vi "Write Scale Scale Fit.vi"(6 "Control Ref Queue":T1, 8 "error in (no error)":errorcluster, 9 "Index":i32, 10 "Scale Fit":u8, 11 "2D Plot.lvclass in":refnum<class "2D Plot.lvclass">) -> (0 "error out":errorcluster, 3 "2D Plot.lvclass out":refnum<class "2D Plot.lvclass">)   [LabVIEW 2017, in "2D Plot.lvclass"]
uses:
  <vilib>/Math Plots/2D Math Plots/2D Plot/2D Plot/2D Plot.lvclass
  <vilib>/Math Plots/2D Math Plots/2D Plot/Action String/2DMathPlot Ctrl Act Queue.ctl
  <vilib>/Math Plots/2D Math Plots/2D Plot/Action String/2DMathPlot Ctrl Act Cluster.ctl
  <vilib>/Math Plots/2D Math Plots/2D Plot/Action String/2DMathPlot State Class.ctl
  <vilib>/Math Plots/2D Math Plots/2D Plot/2D Plot/2D Plot.lvclass/2D Plot.ctl
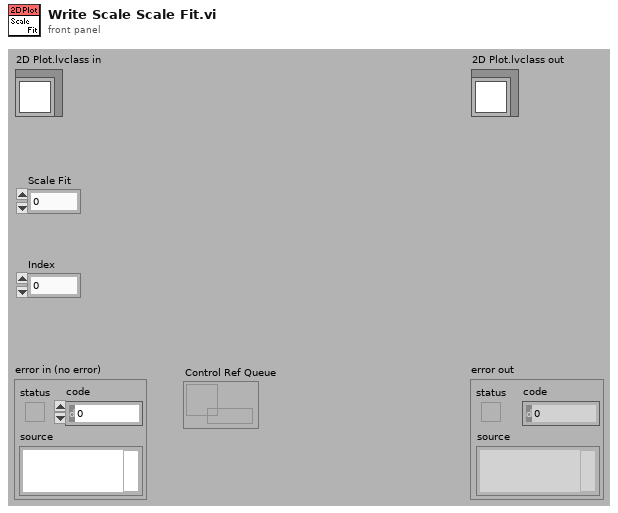
[diagram p1: front panel]
types:
  T1 = typedef "2DMathPlot Ctrl Act Queue.ctl" = refnum<queue>
  T2 = typedef "2D Plot.lvclass/Scale Array.ctl" = T3[]
  T3 = typedef "2D Plot.lvclass/Scale Cluster.ctl" = cluster{"General":cluster{"Editable":bool, "Flipped":bool, "Mapping Mode":u8, "Visible":bool, "Style":u8, "Scale Fit":u8}, "Offset and Multiplier":T4, "Range":cluster{"Minimum":dbl, "Maximum":dbl, "Increment":dbl, "Minor Increment":dbl, "Start":dbl}, "Tick Color":cluster{"Major Color":u32, "Minor Color":u32}, "Gird Color":cluster{"Major Color":u32, "Minor Color":u32}, "Marker":cluster{"Visible":bool, "FG Color":u32, "BG Color":u32, "Font Name":string, "Font Size":u32, "Font Bold":bool, "Font Italic":bool, "Font Strikeout":bool, "Font Underline":bool}, "Name Label":cluster{"Visible":bool, "FG Color":u32, "BG Color":u32, "Font Name":string, "Font Size":u32, "Font Bold":bool, "Font Italic":bool, "Font Strikeout":bool, "Font Underline":bool, "Justification":enum16{"Left", "Center", "Right"}, "Text":string}}
  T4 = typedef "LVOffsetAndMultiplierTypeDef.ctl" = cluster{"Offset":dbl, "Multiplier":dbl}
  T5 = typedef "2DMathPlot Ctrl Act Cluster.ctl" = cluster{"Plot Area Ref":refnum<vi>, "Z Axis Ref":refnum<vi>, "Legend Ref":refnum<vi>, "XControl Ref":refnum<vi>, "Facade Ref":refnum<vi>, "Display State Change Class":T6}
  T6 = typedef "2DMathPlot State Class.ctl" = enum16{"Update All (Undo)", "Update General", "Update Appearance", "Update Format", "Update Scale", "Update Marker", "Update Cursor", "None"}
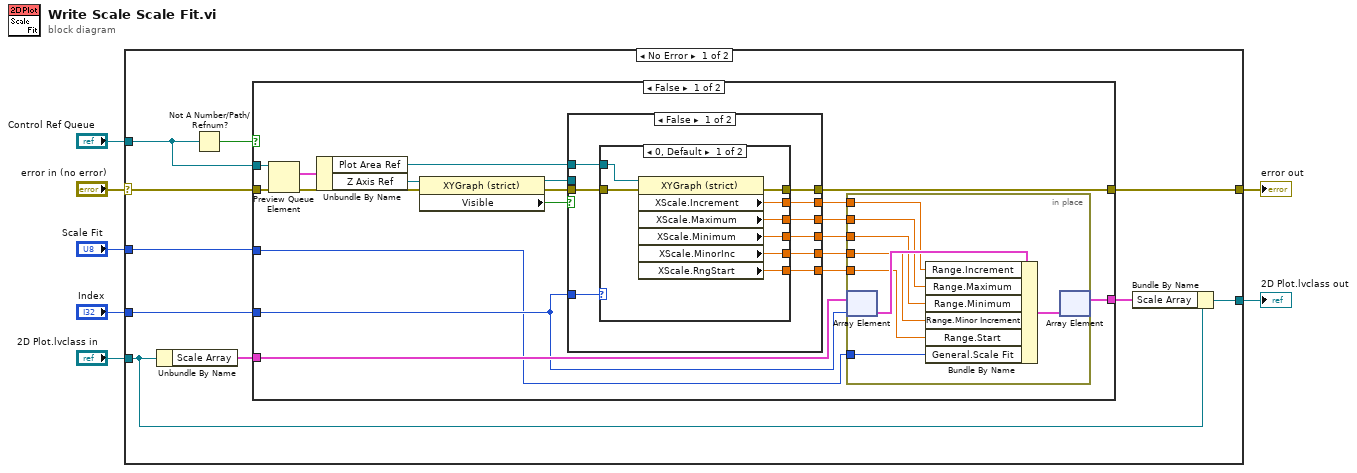
[diagram p0: block diagram]
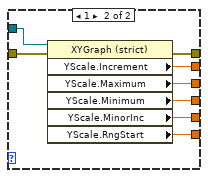
[diagram p2: hidden frame]
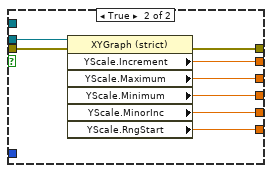
[diagram p3: hidden frame]
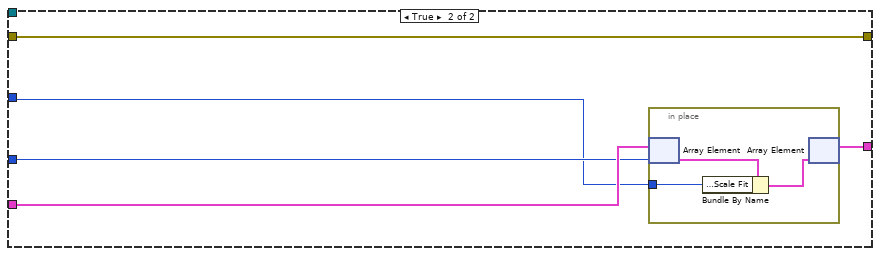
[diagram p4: hidden frame]
diagram:
  n1 = case shown="No Error" "error in (no error)" {
    selector: "error in (no error)" -> [w11 w87]
    tunnel: "2D Plot.lvclass in" -> [w17 w86]
    tunnel: [w16 w86] -> w2
    tunnel: "Control Ref Queue" -> [w9 _]
    tunnel: [w13 w87] -> w1
    tunnel: "Index" -> [w12 _]
    tunnel: "Scale Fit" -> [w10 _]
    frame No Error {
      n2 = Unbundle By Name(w17) -> ("Scale Array"=w15:T2)
      n3 = Not A Number/Path/Refnum?(number/path/refnum=w9) -> (NaN/Path/Refnum?=w8:bool)
      n4 = case shown="False" w8 {
        tunnel: w9 -> [w36 _]
        tunnel: w15 -> [w29 w80]
        tunnel: [w28 w81] -> w14
        tunnel: [w27 w82] -> w13
        tunnel: w12 -> [w21 w79]
        tunnel: w11 -> [w20 w82]
        tunnel: w10 -> [w19 w78]
        frame False {
          n5 = Preview Queue Element(queue=w36, error in (no error)=w20) -> (element=w35:T5, error out=w33:errorcluster)  [unwired: 1 in, 2 out]
          n6 = Unbundle By Name(w35) -> ("Plot Area Ref"=w32:refnum<vi>, "Z Axis Ref"=w18:refnum<vi>)
          n7 = property class="XYGraph (strict)"(reference=w18, error in=w33) -> (reference out=w31:refnum<vi>, error out=w30:errorcluster, "Visible"=w34:bool)
          n8 = case shown="False" w34 {
            tunnel: w30 -> [w53 w76]
            tunnel: [w52 w75] -> w27
            tunnel: w32 -> [w51 _]
            tunnel: w31 -> [_ w77]
            tunnel: [w50 w74] -> w26
            tunnel: [w49 w73] -> w25
            tunnel: [w48 w72] -> w24
            tunnel: [w47 w71] -> w23
            tunnel: [w46 w70] -> w22
            tunnel: w21 -> [w45 _]
            frame False {
              n9 = case shown="0, Default" w45 {
                tunnel: w53 -> [w60 w68]
                tunnel: [w59 w67] -> w52
                tunnel: w51 -> [w61 w69]
                tunnel: [w58 w66] -> w50
                tunnel: [w57 w65] -> w49
                tunnel: [w56 w64] -> w48
                tunnel: [w55 w63] -> w47
                tunnel: [w54 w62] -> w46
                frame 0, Default {
                  n10 = property class="XYGraph (strict)"(reference=w61, error in=w60) -> (error out=w59:errorcluster, "XScale.Increment"=w58:dbl, "XScale.Maximum"=w57:dbl, "XScale.Minimum"=w56:dbl, "XScale.MinorInc"=w55:dbl, "XScale.RngStart"=w54:dbl)  [unwired: 1 out]
                }
                frame 1 {
                  n11 = property class="XYGraph (strict)"(reference=w69, error in=w68) -> (error out=w67:errorcluster, "YScale.Increment"=w66:dbl, "YScale.Maximum"=w65:dbl, "YScale.Minimum"=w64:dbl, "YScale.MinorInc"=w63:dbl, "YScale.RngStart"=w62:dbl)  [unwired: 1 out]
                }
              }
            }
            frame True {
              n12 = property class="XYGraph (strict)"(reference=w77, error in=w76) -> (error out=w75:errorcluster, "YScale.Increment"=w74:dbl, "YScale.Maximum"=w73:dbl, "YScale.Minimum"=w72:dbl, "YScale.MinorInc"=w71:dbl, "YScale.RngStart"=w70:dbl)  [unwired: 1 out]
            }
          }
          n13 = in-place {
            in-place-border: w26 -> [w42]
            in-place-border: w25 -> [w41]
            in-place-border: w24 -> [w40]
            in-place-border: w23 -> [w39]
            in-place-border: w22 -> [w38]
            in-place-border: w19 -> [w37]
            n14 = in-place-array #1(w29, w21) -> (w44:T3)
            n15 = Bundle By Name(cluster=w44, "Range.Increment"=w42, "Range.Maximum"=w41, "Range.Minimum"=w40, "Range.Minor Increment"=w39, "Range.Start"=w38, "General.Scale Fit"=w37) -> (w43:T3)
            n16 = in-place-array #1(w43) -> (w28:T2)  [unwired: 1 out]
          }
        }
        frame True {
          n17 = in-place {
            in-place-border: w78 -> [w83]
            n18 = in-place-array #2(w80, w79) -> (w85:T3)
            n19 = Bundle By Name(cluster=w85, "General.Scale Fit"=w83) -> (w84:T3)
            n20 = in-place-array #2(w84) -> (w81:T2)  [unwired: 1 out]
          }
        }
      }
      n21 = Bundle By Name(cluster=w17, "Scale Array"=w14) -> (w16:refnum<class "2D Plot.lvclass">)
    }
    frame Error {
    }
  }
  "error out" <- w1
  "2D Plot.lvclass out" <- w2
